vi "Constants.vi"() -> (0 "Cp of FLiNaK (J/kgK)":dbl=1883.0, 1 "Cp of Air (J/kgK)":dbl=1007.0, 6 "MHX Tube Pitch (m)":dbl, 7 "Sec Loop Width (m)":dbl, 8 "Thermal Conductivity of Hastealloy N (W/m-K)":dbl, 9 "MHX Tube Diameter (m)":dbl, 10 "Pipe Diameter (m)":dbl, 11 "Dctl (m)":dbl, 12 "Stack Height (m)":dbl, 13 "Sec Loop Height (m)":dbl, 14 "Thermal Conductivity of FLiNaK (W/m-K)":dbl, 15 "MHX Length (m)":dbl, 16 "NDHX Tube Pitch (m)":dbl, 17 "Number of MHX Baffles":dbl, 18 "Specific Heat Capacity of FLiBe (W/m-K)":dbl, 19 "MHX Tube Wall Thickness (m)":dbl, 20 "NDHX Tube Diameter (m)":dbl, 21 "Thermal Conductivity of FLiBe (W/m-K)":dbl, 22 "NDHX Tube Length (m)":dbl, 23 "MHX Number of Tubes":dbl, 24 "Stack Inner Diameter":dbl, 25 "Pipe X-SectionArea (m^2)":dbl, 26 "NDHX Number of Tubes":dbl)   [LabVIEW 2019]
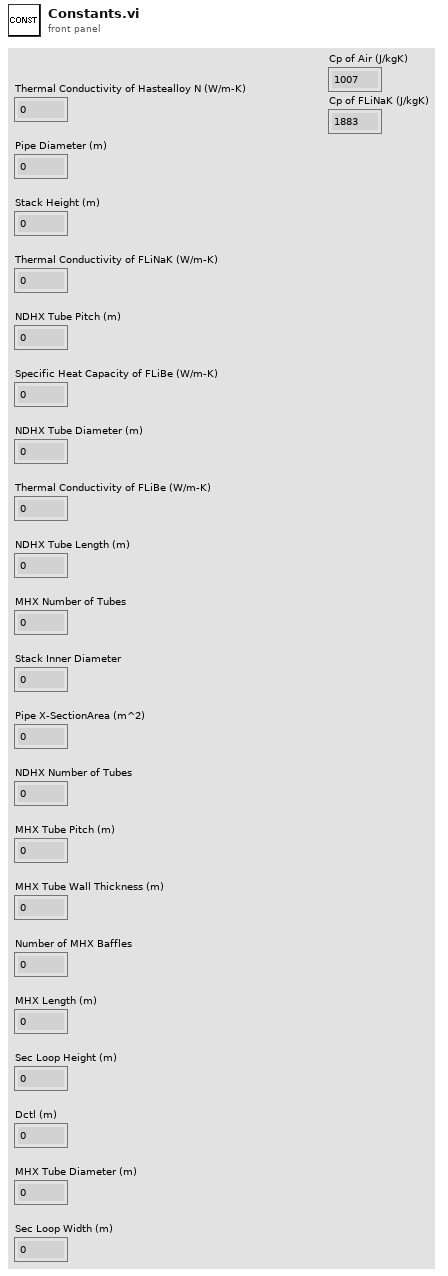
[diagram p1: front panel]
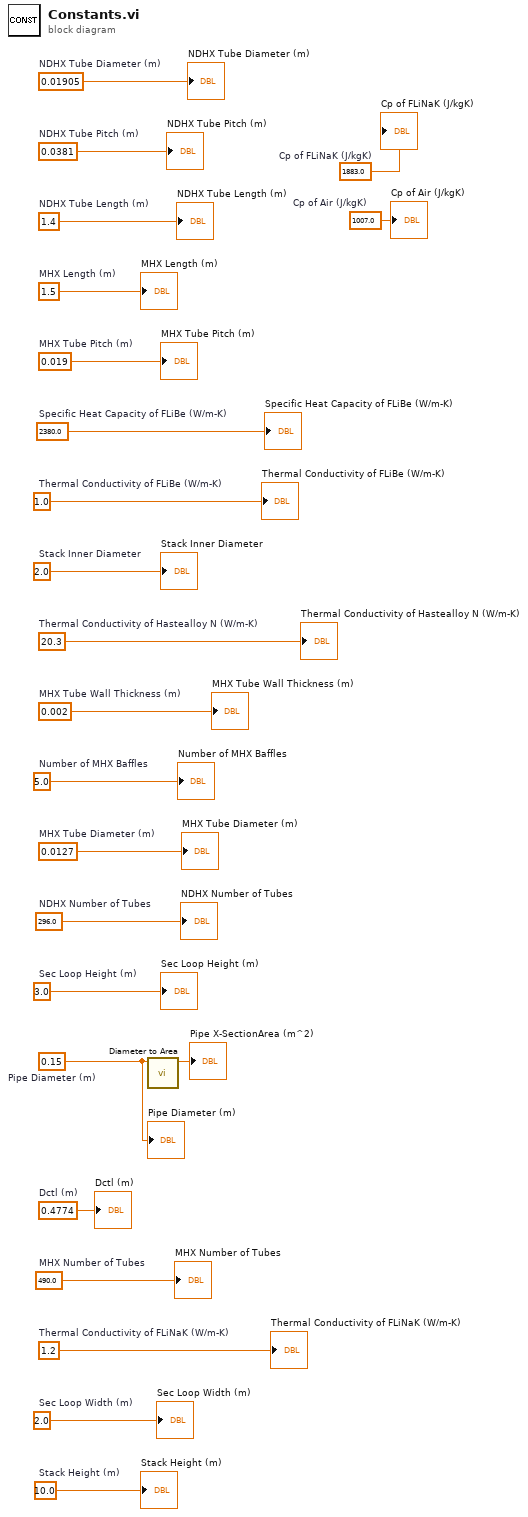
[diagram p0: block diagram]
diagram:
  w2 = 1007.0  # Cp of Air (J/kgK)
  w1 = 1883.0  # Cp of FLiNaK (J/kgK)
  w22 = 490.0  # MHX Number of Tubes
  w18 = 0.002  # MHX Tube Wall Thickness (m)
  w17 = 1.0  # Thermal Conductivity of FLiBe (W/m-K)
  w15 = 2380.0  # Specific Heat Capacity of FLiBe (W/m-K)
  w11 = 5.0  # Number of MHX Baffles
  w10 = 0.4774  # Dctl (m)
  w7 = 0.019  # MHX Tube Pitch (m)
  w23 = 0.0127  # MHX Tube Diameter (m)
  w21 = 1.5  # MHX Length (m)
  w12 = 2.0  # Sec Loop Width (m)
  w13 = 3.0  # Sec Loop Height (m)
  w19 = 20.3  # Thermal Conductivity of Hastealloy N (W/m-K)
  w16 = 1.2  # Thermal Conductivity of FLiNaK (W/m-K)
  w20 = 0.15  # Pipe Diameter (m)
  w5 = 2.0  # Stack Inner Diameter
  w8 = 1.4  # NDHX Tube Length (m)
  w6 = 296.0  # NDHX Number of Tubes
  w3 = 0.0381  # NDHX Tube Pitch (m)
  w9 = 0.01905  # NDHX Tube Diameter (m)
  w4 = 10.0  # Stack Height (m)
  n1 = call "Diameter to Area.vi"("Diameter (m)"=w20) -> ("Area (m^2)"=→"Pipe X-SectionArea (m^2)":dbl)  [unwired: 10 in]
  "MHX Tube Diameter (m)" <- w23
  "MHX Number of Tubes" <- w22
  "MHX Length (m)" <- w21
  "Pipe Diameter (m)" <- w20
  "Thermal Conductivity of Hastealloy N (W/m-K)" <- w19
  "MHX Tube Wall Thickness (m)" <- w18
  "Thermal Conductivity of FLiBe (W/m-K)" <- w17
  "Thermal Conductivity of FLiNaK (W/m-K)" <- w16
  "Specific Heat Capacity of FLiBe (W/m-K)" <- w15
  "Sec Loop Height (m)" <- w13
  "Sec Loop Width (m)" <- w12
  "Number of MHX Baffles" <- w11
  "Dctl (m)" <- w10
  "NDHX Tube Diameter (m)" <- w9
  "NDHX Tube Length (m)" <- w8
  "MHX Tube Pitch (m)" <- w7
  "NDHX Number of Tubes" <- w6
  "Stack Inner Diameter" <- w5
  "Stack Height (m)" <- w4
  "NDHX Tube Pitch (m)" <- w3
  "Cp of Air (J/kgK)" <- w2
  "Cp of FLiNaK (J/kgK)" <- w1
